vi "ElevatorSlow.vi"() -> ()   [LabVIEW 2018]
uses:
  <vilib>/Rock Robotics/WPI/ThirdParty/Phoenix-LabVIEW/Motor Controller/Controls/CTRE_Phoenix_MotorControl_ControlMode.ctl
panel:
  in  "HorsePower":dbl format="%#_13g"
  in  "EncoderValue 2":dbl
  in  "LowerDangerZone 2":dbl
  in  "LowerDangerZone":dbl
  in  "EncoderValue":dbl
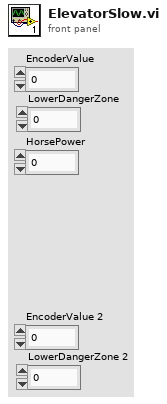
[diagram p1: front panel]
types:
  T1 = typedef "CTRE_Phoenix_MotorControl_ControlMode.ctl" = u16
  T2 = typedef "WPI_MotorControlDeviceRef.ctl" = cluster{"DeviceStatus":errorcluster, "Type":T3, "PWM":cluster{"PWM Channel":T4, "DeadBand":T5}, "CAN":cluster{"Device Number":u8, "SetOutput VI Ref":variant, "GetOutput VI Ref":variant, "Enable VI Ref":variant, "Disable VI Ref":variant, "Data":variant}, "Invert":bool, "DIO PWM":cluster{"PWM \"Enable\" Channel":T4, "DIOChannel":T6, "PWM Rate":dbl}}
  T3 = typedef "WPI_MotorControlType.ctl" = enum16{"PWM", "CAN", "DIO PWM"}
  T4 = typedef "FPGA_DIOPWMChannel.ctl" = enum8{"PWM 0", "PWM 1", "PWM 2", "PWM 3", "PWM 4", "PWM 5", "PWM 6", "PWM 7", "PWM 8", "PWM 9", "PWM MXP 0", "PWM MXP 1", "PWM MXP 2", "PWM MXP 3", "PWM MXP 4", "PWM MXP 5", "PWM MXP 6", "PWM MXP 7", "PWM MXP 8", "PWM MXP 9", "Invalid"}
  T5 = typedef "WPI_PWMDeadband.ctl" = cluster{"Name":string, "maxPositivePwm":i32, "minPositivePwm":i32, "centerPwm":i32, "maxNegativePwm":i32, "minNegativePwm":i32, "angularRange":u16}
  T6 = typedef "FPGA_DIOChannel.ctl" = enum8{"DIO 0", "DIO 1", "DIO 2", "DIO 3", "DIO 4", "DIO 5", "DIO 6", "DIO 7", "DIO 8", "DIO 9", "DIO MXP 0", "DIO MXP 1", "DIO MXP 2", "DIO MXP 3", "DIO MXP 4", "DIO MXP 5", "DIO MXP 6", "DIO MXP 7", "DIO MXP 8", "DIO MXP 9", "DIO MXP 10", "DIO MXP 11", "DIO MXP 12", "DIO MXP 13", "DIO MXP 14", "DIO MXP 15", "SPI Port CS1", "SPI Port CS2", "SPI Port CS3", "SPI Port MISO", "SPI Port MOSI", "Invalid"}
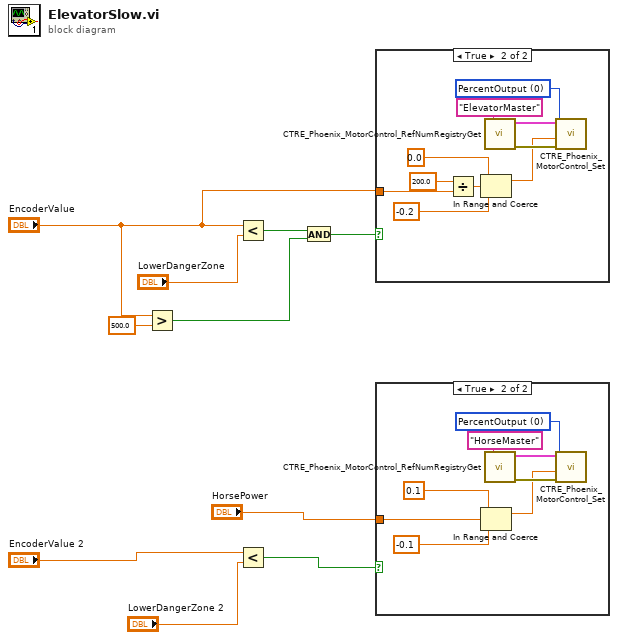
[diagram p0: block diagram]
diagram:
  n1 = Greater?(x="EncoderValue", y=500.0) -> (0:w5:bool)
  n2 = Less?(x="EncoderValue", y="LowerDangerZone") -> (x < y?=w9:bool)
  n3 = Less?(x="EncoderValue 2", y="LowerDangerZone 2") -> (x < y?=w2:bool)
  n4 = And(x=w9, y=w5) -> (x .and. y?=w8:bool)
  n5 = case shown="True" w8 {
    tunnel: "EncoderValue" -> [_ w16]
    frame False {
    }
    frame True {
      w17 = T1 0 items=["PercentOutput"=0, "Position"=1, "Velocity"=2, "Current"=3, "Follower"=5, "MotionProfile"=6, "MotionMagic"=7, "MotionProfileArc"=10, "Disabled"=15] ("Control Mode")
      n6 = Divide(x=200.0, y=w16) -> (x/y=w14:dbl)
      n7 = In Range and Coerce(upper limit=0.0, x=w14, lower limit=-0.2) -> (coerced(x)=w11:dbl)  [unwired: 1 out]
      n8 = call <vilib>:"CTRE_Phoenix_MotorControl_RefNumRegistryGet.vi"("refnum name"="ElevatorMaster") -> ("error out"=w18:errorcluster, "PhoenixMotorControlDevRef"=w19:T2)  [unwired: 9 in]
      n9 = call <vilib>:"CTRE_Phoenix_MotorControl_Set.vi"("error in (no error)"=w18, "Output"=w11, "Control Mode"=w17, "PhoenixMotorControlDevRef"=w19) -> ()  [unwired: 6 in, 2 out]
    }
  }
  n10 = case shown="True" w2 {
    tunnel: "HorsePower" -> [_ w21]
    frame False {
    }
    frame True {
      w25 = T1 0 items=["PercentOutput"=0, "Position"=1, "Velocity"=2, "Current"=3, "Follower"=5, "MotionProfile"=6, "MotionMagic"=7, "MotionProfileArc"=10, "Disabled"=15] ("Control Mode")
      n11 = In Range and Coerce(upper limit=0.1, x=w21, lower limit=-0.1) -> (coerced(x)=w22:dbl)  [unwired: 1 out]
      n12 = call <vilib>:"CTRE_Phoenix_MotorControl_RefNumRegistryGet.vi"("refnum name"="HorseMaster") -> ("error out"=w26:errorcluster, "PhoenixMotorControlDevRef"=w27:T2)  [unwired: 9 in]
      n13 = call <vilib>:"CTRE_Phoenix_MotorControl_Set.vi"("error in (no error)"=w26, "Output"=w22, "Control Mode"=w25, "PhoenixMotorControlDevRef"=w27) -> ()  [unwired: 6 in, 2 out]
    }
  }
